vi "remove from flattened hierarchy.vi"(8 "error in":errorcluster, 10 "NISE_CEF_serializable configuration in":T1, 11 "memory hierarchy in":T2) -> (0 "error out":errorcluster, 3 "memory hierarchy out":T2)   [LabVIEW 2013, in "NISE_CEF_TreeSerializer.lvlib"]
doc: "Removes a flattened configuration from a flattened instance set, along with all children. This function only uses the ID field at present."
uses:
  NISE_CEF_TreeSerializer.lvlib
  flat hierarchy.ctl
  full hierarchy.ctl
  hierarchy element.ctl
  instance data.ctl
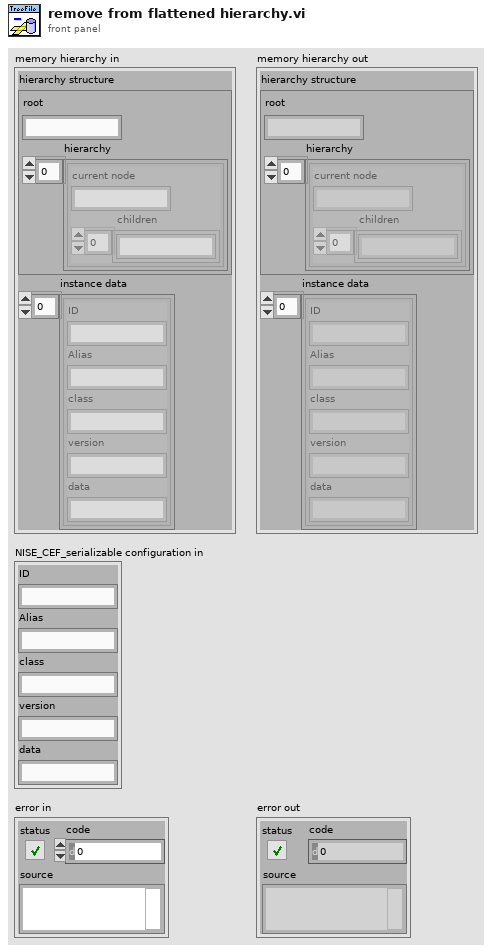
[diagram p1: front panel]
types:
  T1 = typedef "NISE_CEF_TreeSerializer.lvlib/instance data.ctl" = cluster{"ID":string, "Alias":string, "class":string, "version":string, "data":string}
  T2 = typedef "NISE_CEF_TreeSerializer.lvlib/flat hierarchy.ctl" = cluster{"hierarchy structure":T3, "instance data":T1[]}
  T3 = typedef "NISE_CEF_TreeSerializer.lvlib/full hierarchy.ctl" = cluster{"root":string, "hierarchy":T4[]}
  T4 = typedef "NISE_CEF_TreeSerializer.lvlib/hierarchy element.ctl" = cluster{"current node":string, "children":string[]}
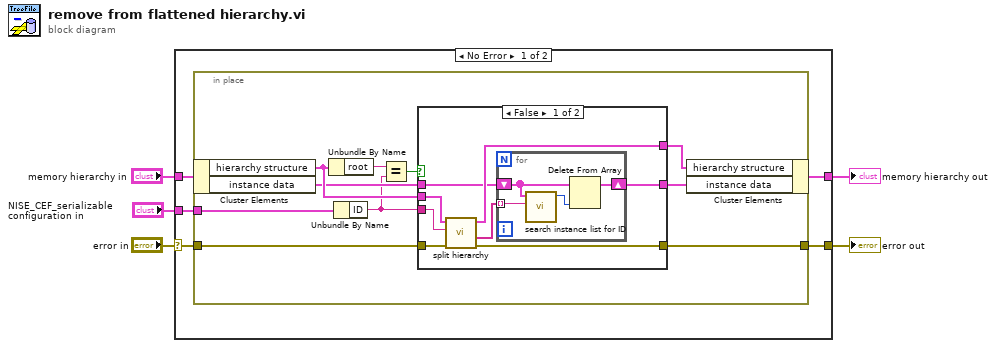
[diagram p0: block diagram]
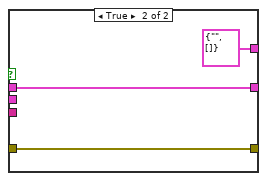
[diagram p2: hidden frame]
diagram:
  n1 = case shown="No Error" "error in" {
    selector: "error in" -> [w7 w37]
    tunnel: [w10 w36] -> w5
    tunnel: "memory hierarchy in" -> [w9 w36]
    tunnel: "NISE_CEF_serializable configuration in" -> [w8 _]
    tunnel: [w6 w37] -> w1
    frame No Error {
      n2 = in-place {
        in-place-border: w8 -> [w11]
        in-place-border: w7 -> [w14]
        in-place-border: [w13] -> w6
        n3 = in-place-cluster #1(w9) -> ("hierarchy structure"=w20:T3, "instance data"=w16:T1[])
        n4 = Unbundle By Name(w20) -> ("root"=w19:string)
        n5 = Unbundle By Name(w11) -> ("ID"=w12:string)
        n6 = Equal?(x=w19, y=w12) -> (x = y?=w18:bool)
        n7 = case shown="False" w18 {
          tunnel: w20 -> [w28 _]
          tunnel: [w25 T3 {"root"="", "hierarchy"=[]} ("hierarchy structure")] -> w17
          tunnel: w16 -> [w22 w34]
          tunnel: [w21 w34] -> w15
          tunnel: w14 -> [w27 w33]
          tunnel: [w26 w33] -> w13
          tunnel: w12 -> [w24 _]
          frame False {
            n8 = call "split hierarchy.vi"("error in"=w27, "UID to split"=w24, "hierarchy structure"=w28) -> ("error out"=w26:errorcluster, "UIDs moved"=w23:string[], "hierarchy excluding UID"=w25:T3)  [unwired: 5 in, 1 out]
            n9 = for {
              tunnel: w23 -> [w29] mode=indexing
              shift-right: [w31] -> w21
              shift-left: w22 -> [w32]
              n10 = call "search instance list for ID.vi"("UID"=w29, "instance data"=w32) -> ("index"=w30:i32)  [unwired: 9 in]
              n11 = Delete From Array(array=w32, index=w30) -> (array with subset deleted=w31:T1[])  [unwired: 1 in, 1 out]
            }
          }
          frame True {
          }
        }
        n12 = in-place-cluster #1("hierarchy structure"=w17, "instance data"=w15) -> (w10:T2)
      }
    }
    frame Error {
    }
  }
  "memory hierarchy out" <- w5
  "error out" <- w1
